vi "Write Anything.vi"(0 "refnum":T1, 5 "user parameter references in":refnum<vi>[](array[refnum]), 11 "error in":errorcluster, 12 "additional information":string) -> (4 "refnum out":T1, 15 "error out":errorcluster)   [LabVIEW 2018, in "Springboard TLB`.lvlib" / "Springboard TLB`.lvclass"]
uses:
  Springboard TLB`.lvclass
  <vilib>/Utility/config.llb/Config Data RefNum.ctl
  <vilib>/Utility/error.llb/Error Cluster From Error Code.vi
  <vilib>/Utility/config.llb/Write Key (String).vi
  <vilib>/ErrorRing/Error Ring.xnode
  <vilib>/Utility/config.llb/NI_LVConfig.lvlib
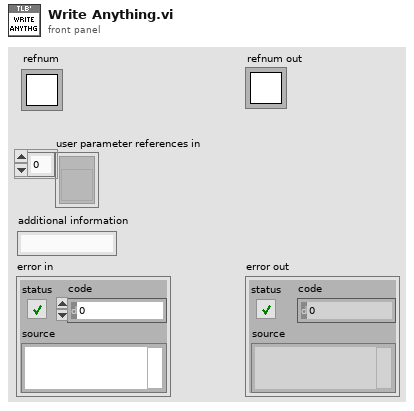
[diagram p1: front panel]
types:
  T1 = typedef "NI_LVConfig.lvlib/Config Data RefNum.ctl" = refnum<k1>
  T2 = typedef "LVNumericRepresentation.ctl" = enum32{"Extended Precision", "Double Precision", "Single Precision", "Long", "Word", "Byte", "Unsigned Long", "Unsigned Word", "Unsigned Byte", "Complex Extended", "Complex Double", "Complex Single", "Quad", "Unsigned Quad", "Fixed-Point"}
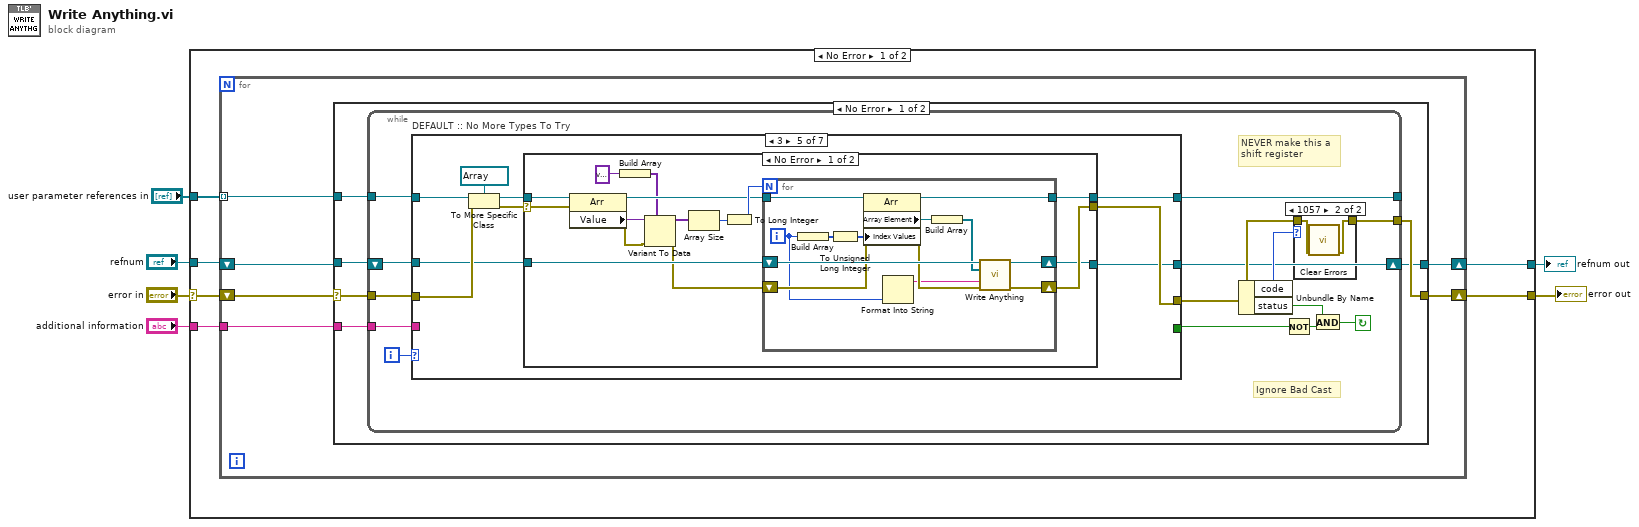
[diagram p0: block diagram]
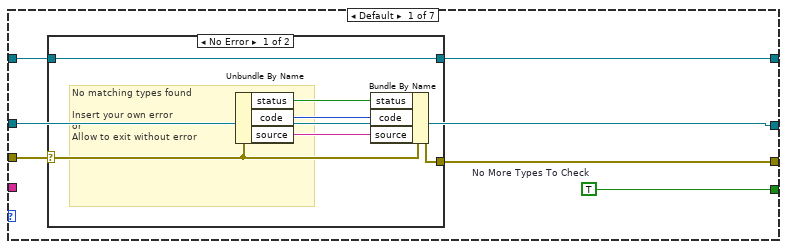
[diagram p2: hidden frame]
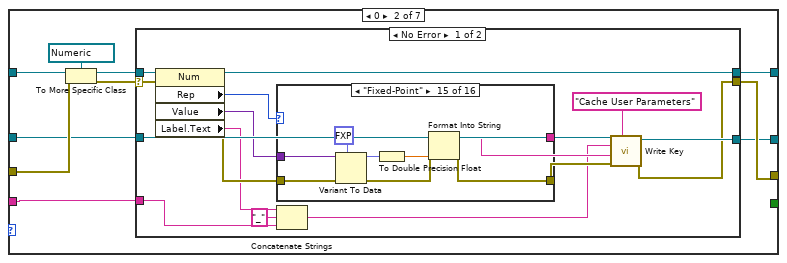
[diagram p4: hidden frame]
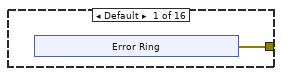
[diagram p5: hidden frame]
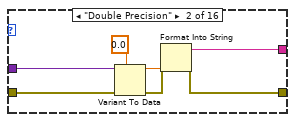
[diagram p6: hidden frame]
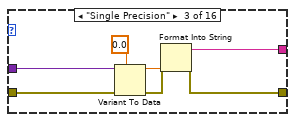
[diagram p7: hidden frame]
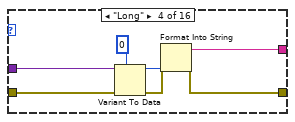
[diagram p8: hidden frame]
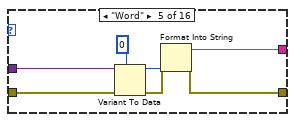
[diagram p9: hidden frame]
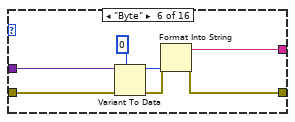
[diagram p10: hidden frame]
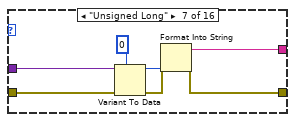
[diagram p11: hidden frame]
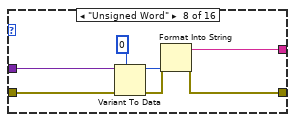
[diagram p12: hidden frame]
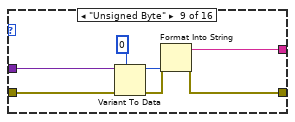
[diagram p13: hidden frame]
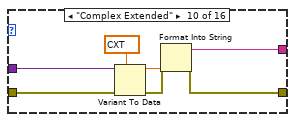
[diagram p14: hidden frame]
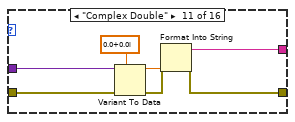
[diagram p15: hidden frame]
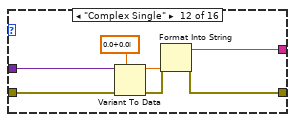
[diagram p16: hidden frame]
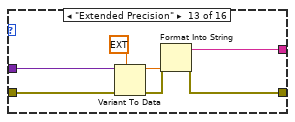
[diagram p17: hidden frame]
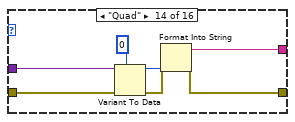
[diagram p18: hidden frame]
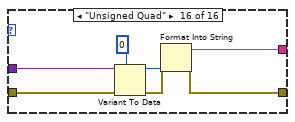
[diagram p19: hidden frame]
diagram:
  n1 = case shown="No Error" "error in" {
    selector: "error in" -> [w10 w346]
    tunnel: "user parameter references in" -> [w12 _]
    tunnel: [w11 w346] -> w4
    tunnel: "refnum" -> [w9 w345]
    tunnel: [w8 w345] -> w2
    tunnel: "additional information" -> [w7 _]
    frame No Error {
      n2 = for {
        tunnel: w12 -> [w16] mode=indexing
        shift-right: [w18] -> w11
        shift-left: w10 -> [w17]
        shift-right: [w15] -> w8
        shift-left: w9 -> [w14]
        tunnel: w7 -> [w13]
        n3 = case shown="No Error" w17 {
          selector: w17 -> [w23 w344]
          tunnel: w16 -> [w24 _]
          tunnel: [w22 w344] -> w18
          tunnel: w14 -> [w21 w343]
          tunnel: [w20 w343] -> w15
          tunnel: w13 -> [w19 _]
          frame No Error {
            n4 = while {
              tunnel: w24 -> [w34]
              tunnel: w23 -> [w32]
              tunnel: [w29] -> _
              tunnel: [w28] -> w22
              shift-right: [w26] -> w20
              shift-left: w21 -> [w27]
              tunnel: w19 -> [w25]
              i -> [w33]
              stop <- w35 continue-if-true
              # "NEVER make this a\nshift register"
              # "Ignore Bad Cast"
              n5 = case "DEFAULT :: No More Types To Try" shown="3" w33 {
                tunnel: w32 -> [w41 w62 w203 w230 w251 w291 w317]
                tunnel: w34 -> [w42 w60 w201 w228 w249 w289 w315]
                tunnel: [w43 w56 w197 w224 w245 w285 w311] -> w29
                tunnel: [w40 w57 w198 w225 w246 w286 w312] -> w31
                tunnel: [w44 _ _ _ _ _ _] -> w30
                tunnel: w27 -> [w39 w55 w196 w223 w244 w284 w310]
                tunnel: [w39 w54 w195 w222 w243 w283 w309] -> w26
                tunnel: w25 -> [_ w53 w194 w221 _ w282 w308]
                frame Default {
                  w44 = TRUE  # No More Types To Check
                  n6 = case shown="No Error" w41 {
                    selector: w41 -> [w48 w51]
                    tunnel: [w50 w52] -> w43
                    tunnel: w42 -> [w50 w52]
                    tunnel: [w49 w51] -> w40
                    frame No Error {
                      # "No matching types found\n\nInsert your own error \nor\nAllow to exit without error"
                      n7 = Unbundle By Name(w48) -> ("status"=w47:bool, "code"=w46:i32, "source"=w45:string)
                      n8 = Bundle By Name(cluster=w48, "status"=w47, "code"=w46, "source"=w45) -> (w49:errorcluster)
                    }
                    frame Error {
                      # "No matching types found\n\nAllow this non-typecast error to propogate through without modification"
                    }
                  }
                }
                frame 0 {
                  n9 = To More Specific Class(target class=refnum<vi> refnum ("Waveform Chart"), reference=w60, error in=w62) -> (specific class reference=w59:refnum<vi>, error out=w58:errorcluster)
                  n10 = case shown="No Error" w58 {
                    selector: w58 -> [w77 w193]
                    tunnel: w59 -> [w78 w192]
                    tunnel: [w70 w193] -> w57
                    tunnel: [w76 w192] -> w56
                    tunnel: w55 -> [w74 w191]
                    tunnel: [w73 w191] -> w54
                    tunnel: w53 -> [w64 _]
                    frame No Error {
                      n11 = property class="Num"(reference=w78, error in=w77) -> (reference out=w76:refnum<vi>, error out=w72:errorcluster, "Rep"=w68:T2, "Value"=w69:variant, "Label.Text"=w66:string)
                      n12 = case shown="\"Fixed-Point\"" w68 {
                        tunnel: w72 -> [_ w91 w98 w105 w112 w119 w126 w133 w140 w147 w154 w161 w168 w175 w183 w190]
                        tunnel: [w79 w86 w93 w100 w107 w114 w121 w128 w135 w142 w149 w156 w163 w170 w178 w185] -> w71
                        tunnel: w69 -> [_ w90 w97 w104 w111 w118 w125 w132 w139 w146 w153 w160 w167 w174 w182 w189]
                        tunnel: [_ w85 w92 w99 w106 w113 w120 w127 w134 w141 w148 w155 w162 w169 w177 w184] -> w67
                        frame Default {
                          n13 = xnode "Error Ring"() -> ("error out"=w79:errorcluster)
                        }
                        frame "Double Precision" {
                          n14 = Variant To Data(error in=w91, type=0.0, Variant=w90) -> (data=w88:dbl, error out=w87:errorcluster)
                          n15 = Format Into String(error in=w87, w88) -> (resulting string=w85:string, error out=w86:errorcluster)  [unwired: 2 in]
                        }
                        frame "Single Precision" {
                          n16 = Variant To Data(error in=w98, type=sgl 0.0, Variant=w97) -> (data=w95:sgl, error out=w94:errorcluster)
                          n17 = Format Into String(error in=w94, w95) -> (resulting string=w92:string, error out=w93:errorcluster)  [unwired: 2 in]
                        }
                        frame "Long" {
                          n18 = Variant To Data(error in=w105, type=0, Variant=w104) -> (data=w102:i32, error out=w101:errorcluster)
                          n19 = Format Into String(error in=w101, w102) -> (resulting string=w99:string, error out=w100:errorcluster)  [unwired: 2 in]
                        }
                        frame "Word" {
                          n20 = Variant To Data(error in=w112, type=i16 0, Variant=w111) -> (data=w109:i16, error out=w108:errorcluster)
                          n21 = Format Into String(error in=w108, w109) -> (resulting string=w106:string, error out=w107:errorcluster)  [unwired: 2 in]
                        }
                        frame "Byte" {
                          n22 = Variant To Data(error in=w119, type=i8 0, Variant=w118) -> (data=w116:i8, error out=w115:errorcluster)
                          n23 = Format Into String(error in=w115, w116) -> (resulting string=w113:string, error out=w114:errorcluster)  [unwired: 2 in]
                        }
                        frame "Unsigned Long" {
                          n24 = Variant To Data(error in=w126, type=u32 0, Variant=w125) -> (data=w123:u32, error out=w122:errorcluster)
                          n25 = Format Into String(error in=w122, w123) -> (resulting string=w120:string, error out=w121:errorcluster)  [unwired: 2 in]
                        }
                        frame "Unsigned Word" {
                          n26 = Variant To Data(error in=w133, type=u16 0, Variant=w132) -> (data=w130:u16, error out=w129:errorcluster)
                          n27 = Format Into String(error in=w129, w130) -> (resulting string=w127:string, error out=w128:errorcluster)  [unwired: 2 in]
                        }
                        frame "Unsigned Byte" {
                          n28 = Variant To Data(error in=w140, type=u8 0, Variant=w139) -> (data=w137:u8, error out=w136:errorcluster)
                          n29 = Format Into String(error in=w136, w137) -> (resulting string=w134:string, error out=w135:errorcluster)  [unwired: 2 in]
                        }
                        frame "Complex Extended" {
                          n30 = Variant To Data(error in=w147, type=cxt 0.0+0.0i, Variant=w146) -> (data=w144:cxt, error out=w143:errorcluster)
                          n31 = Format Into String(error in=w143, w144) -> (resulting string=w141:string, error out=w142:errorcluster)  [unwired: 2 in]
                        }
                        frame "Complex Double" {
                          n32 = Variant To Data(error in=w154, type=cdb 0.0+0.0i, Variant=w153) -> (data=w151:cdb, error out=w150:errorcluster)
                          n33 = Format Into String(error in=w150, w151) -> (resulting string=w148:string, error out=w149:errorcluster)  [unwired: 2 in]
                        }
                        frame "Complex Single" {
                          n34 = Variant To Data(error in=w161, type=csg 0.0+0.0i, Variant=w160) -> (data=w158:csg, error out=w157:errorcluster)
                          n35 = Format Into String(error in=w157, w158) -> (resulting string=w155:string, error out=w156:errorcluster)  [unwired: 2 in]
                        }
                        frame "Extended Precision" {
                          n36 = Variant To Data(error in=w168, type=ext 0.0, Variant=w167) -> (data=w165:ext, error out=w164:errorcluster)
                          n37 = Format Into String(error in=w164, w165) -> (resulting string=w162:string, error out=w163:errorcluster)  [unwired: 2 in]
                        }
                        frame "Quad" {
                          n38 = Variant To Data(error in=w175, type=i64 0, Variant=w174) -> (data=w172:i64, error out=w171:errorcluster)
                          n39 = Format Into String(error in=w171, w172) -> (resulting string=w169:string, error out=w170:errorcluster)  [unwired: 2 in]
                        }
                        frame "Fixed-Point" {
                          n40 = Variant To Data(error in=w183, type=fxp<+,1,1> 0.0, Variant=w182) -> (data=w180:fxp<+,1,1>, error out=w179:errorcluster)
                          n41 = To Double Precision Float(number=w180) -> (double precision float=w176:dbl)
                          n42 = Format Into String(error in=w179, w176) -> (resulting string=w177:string, error out=w178:errorcluster)  [unwired: 2 in]
                        }
                        frame "Unsigned Quad" {
                          n43 = Variant To Data(error in=w190, type=u64 0, Variant=w189) -> (data=w187:u64, error out=w186:errorcluster)
                          n44 = Format Into String(error in=w186, w187) -> (resulting string=w184:string, error out=w185:errorcluster)  [unwired: 2 in]
                        }
                      }
                      n45 = Concatenate Strings(w66, "_" ("string"), w64) -> (w65:string)
                      n46 = call-poly <vilib>:"Write Key.vi"("section"="Cache User Parameters", "error in (no error)"=w71, "value"=w67, "key"=w65, "refnum"=w74) -> ("error out"=w70:errorcluster, "refnum out"=w73:T1)  [unwired: 4 in, 1 out]
                    }
                    frame Error {
                    }
                  }
                }
                frame 1 {
                  n47 = To More Specific Class(target class=refnum<vi> refnum ("Waveform Chart"), reference=w201, error in=w203) -> (specific class reference=w200:refnum<vi>, error out=w199:errorcluster)
                  n48 = case shown="No Error" w199 {
                    selector: w199 -> [w216 w220]
                    tunnel: w200 -> [w217 w219]
                    tunnel: [w210 w220] -> w198
                    tunnel: [w215 w219] -> w197
                    tunnel: w196 -> [w213 w218]
                    tunnel: [w212 w218] -> w195
                    tunnel: w194 -> [w205 _]
                    frame No Error {
                      n49 = property class="Path"(reference=w217, error in=w216) -> (reference out=w215:refnum<vi>, error out=w207:errorcluster, "Label.Text"=w211:string, "Value"=w209:path)
                      n50 = Path To String(path=w209) -> (string=w208:string)
                      n51 = Concatenate Strings(w211, "_" ("string"), w205) -> (w206:string)
                      n52 = call-poly <vilib>:"Write Key.vi"("section"="Cache User Parameters", "error in (no error)"=w207, "value"=w208, "key"=w206, "refnum"=w213) -> ("error out"=w210:errorcluster, "refnum out"=w212:T1)  [unwired: 4 in, 1 out]
                    }
                    frame Error {
                    }
                  }
                }
                frame 2 {
                  n53 = To More Specific Class(target class=refnum<vi> refnum ("Waveform Chart"), reference=w228, error in=w230) -> (specific class reference=w227:refnum<vi>, error out=w226:errorcluster)
                  n54 = case shown="No Error" w226 {
                    selector: w226 -> [w238 w242]
                    tunnel: w227 -> [w239 w241]
                    tunnel: [w234 w242] -> w225
                    tunnel: [w237 w241] -> w224
                    tunnel: w223 -> [w233 w240]
                    tunnel: [w232 w240] -> w222
                    tunnel: w221 -> [w231 _]
                    frame No Error {
                      n55 = property class="Clust"(reference=w239, error in=w238) -> (reference out=w237:refnum<vi>, error out=w235:errorcluster, "Controls[]"=w236:refnum<vi>[])
                      n56 = call "Write Anything.vi"("refnum"=w233, "user parameter references in"=w236, "error in"=w235, "additional information"=w231) -> ("refnum out"=w232:T1, "error out"=w234:errorcluster)  [unwired: 10 in]
                    }
                    frame Error {
                    }
                  }
                }
                frame 3 {
                  n57 = To More Specific Class(target class=refnum<vi> refnum ("Waveform Chart"), reference=w249, error in=w251) -> (specific class reference=w248:refnum<vi>, error out=w247:errorcluster)
                  n58 = case shown="No Error" w247 {
                    selector: w247 -> [w265 w281]
                    tunnel: w248 -> [w266 w280]
                    tunnel: [w264 w281] -> w246
                    tunnel: [w259 w280] -> w245
                    tunnel: w244 -> [w263 w279]
                    tunnel: [w262 w279] -> w243
                    frame No Error {
                      n59 = property class="Arr"(reference=w266, error in=w265) -> (reference out=w260:refnum<vi>, error out=w253:errorcluster, "Value"=w258:variant)
                      n60 = Build Array(variant ("type")) -> (w256:variant[])
                      n61 = Variant To Data(error in=w253, type=w256, Variant=w258) -> (data=w255:variant[], error out=w252:errorcluster)
                      n62 = Array Size(array=w255) -> (size(s)=w254:i32)
                      n63 = To Long Integer(number=w254) -> (32bit integer=w261:i32)
                      n64 = for {
                        N: w261 -> [_]
                        shift-right: [w278] -> w264
                        shift-left: w252 -> [w274]
                        shift-right: [w276] -> w262
                        shift-left: w263 -> [w277]
                        tunnel: w260 -> [w275]
                        tunnel: [w275] -> w259
                        i -> [w267]
                        n65 = Build Array(w267) -> (w273:i32[])
                        n66 = To Unsigned Long Integer(number=w273) -> (unsigned 32bit integer=w269:u32[])
                        n67 = property class="Arr"(reference=w275, error in=w274, "Index Values"=w269) -> (error out=w272:errorcluster, "Array Element"=w271:refnum<vi>)  [unwired: 1 out]
                        n68 = Format Into String(w267) -> (resulting string=w268:string)  [unwired: 3 in, 1 out]
                        n69 = Build Array(w271) -> (w270:refnum<vi>[])
                        n70 = call "Write Anything.vi"("refnum"=w277, "user parameter references in"=w270, "error in"=w272, "additional information"=w268) -> ("refnum out"=w276:T1, "error out"=w278:errorcluster)  [unwired: 10 in]
                      }
                    }
                    frame Error {
                    }
                  }
                }
                frame 4 {
                  n71 = To More Specific Class(target class=refnum<vi> refnum ("Waveform Chart"), reference=w289, error in=w291) -> (specific class reference=w288:refnum<vi>, error out=w287:errorcluster)
                  n72 = case shown="No Error" w287 {
                    selector: w287 -> [w303 w307]
                    tunnel: w288 -> [w304 w306]
                    tunnel: [w297 w307] -> w286
                    tunnel: [w302 w306] -> w285
                    tunnel: w284 -> [w300 w305]
                    tunnel: [w299 w305] -> w283
                    tunnel: w282 -> [w293 _]
                    frame No Error {
                      n73 = property class="Str"(reference=w304, error in=w303) -> (reference out=w302:refnum<vi>, error out=w296:errorcluster, "Label.Text"=w298:string, "Value"=w295:string)
                      n74 = Concatenate Strings(w298, "_" ("string"), w293) -> (w294:string)
                      n75 = call-poly <vilib>:"Write Key.vi"("section"="Cache User Parameters", "error in (no error)"=w296, "value"=w295, "key"=w294, "refnum"=w300) -> ("error out"=w297:errorcluster, "refnum out"=w299:T1)  [unwired: 4 in, 1 out]
                    }
                    frame Error {
                    }
                  }
                }
                frame 5 {
                  n76 = To More Specific Class(target class=refnum<vi> refnum ("Waveform Chart"), reference=w315, error in=w317) -> (specific class reference=w314:refnum<vi>, error out=w313:errorcluster)
                  n77 = case shown="No Error" w313 {
                    selector: w313 -> [w335 w339]
                    tunnel: w314 -> [w336 w338]
                    tunnel: [w327 w339] -> w312
                    tunnel: [w334 w338] -> w311
                    tunnel: w310 -> [w332 w337]
                    tunnel: [w331 w337] -> w309
                    tunnel: w308 -> [w319 _]
                    frame No Error {
                      n78 = property class="Bool"(reference=w336, error in=w335) -> (reference out=w334:refnum<vi>, error out=w330:errorcluster, "Label.Text"=w326:string, "Value"=w329:variant)
                      n79 = Variant To Data(error in=w330, type=TRUE, Variant=w329) -> (data=w324:bool, error out=w328:errorcluster)
                      n80 = Select(t="True" ("section"), s=w324, f="False" ("section")) -> (s? t:f=w321:string)
                      n81 = Concatenate Strings(w326, "_" ("string"), w319) -> (w320:string)
                      n82 = call-poly <vilib>:"Write Key.vi"("section"="Cache User Parameters", "error in (no error)"=w328, "value"=w321, "key"=w320, "refnum"=w332) -> ("error out"=w327:errorcluster, "refnum out"=w331:T1)  [unwired: 4 in, 1 out]
                    }
                    frame Error {
                    }
                  }
                }
              }
              n83 = Unbundle By Name(w31) -> ("code"=w36:i32, "status"=w37:bool)
              n84 = Not(x=w30) -> (.not. x?=w38:bool)
              n85 = case shown="1057" w36 {
                tunnel: [w340 w342] -> w28
                tunnel: w31 -> [w340 w341]
                frame Default {
                }
                frame 1057 {
                  n86 = call <vilib>:"Clear Errors.vi"("error in (no error)"=w341) -> ("error out"=w342:errorcluster)  [unwired: 5 in, 1 out]
                }
              }
              n87 = And(x=w37, y=w38) -> (x .and. y?=w35:bool)
            }
          }
          frame Error {
          }
        }
      }
    }
    frame Error {
    }
  }
  "error out" <- w4
  "refnum out" <- w2
